vi "Rename_drag.vi"(10 "data name":string, 11 "Data":T1(array[cluster])) -> (3 "Array":T1(array[cluster]))   [LabVIEW 2016]
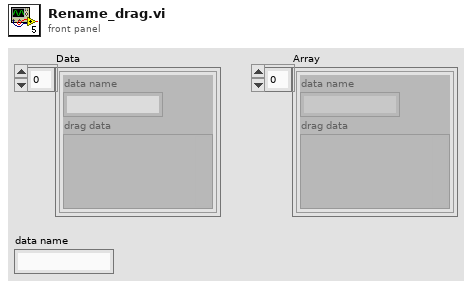
[diagram p1: front panel]
types:
  T1 = cluster{"data name":string, "drag data":variant}[]
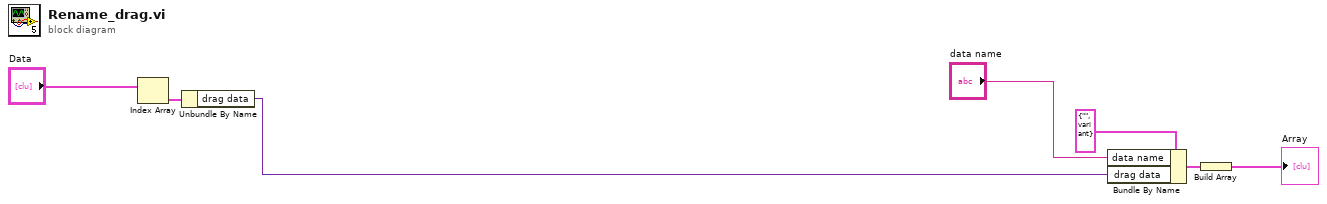
[diagram p0: block diagram]
diagram:
  n1 = Index Array(array="Data") -> (element=w4:cluster{"data name":string, "drag data":variant})  [unwired: 1 in]
  n2 = Unbundle By Name(w4) -> ("drag data"=w5:variant)
  n3 = Bundle By Name(cluster=cluster{"data name":string, "drag data":variant} {"data name"="", "drag data"=variant}, "data name"="data name", "drag data"=w5) -> (w6:cluster{"data name":string, "drag data":variant})
  n4 = Build Array(w6) -> (→"Array":T1)
